vi "Read Address.vi"(8 "error in":errorcluster, 11 "Node in":refnum<class "Node.lvclass">) -> (0 "error out":errorcluster, 2 "Address":i32[](array[numeric]), 3 "Node out":refnum<class "Node.lvclass">)   [LabVIEW 2014, in "Node.lvclass"]
uses:
  Node.lvclass
  Node.lvclass/Node.ctl
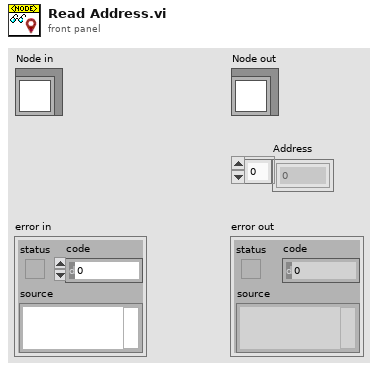
[diagram p1: front panel]
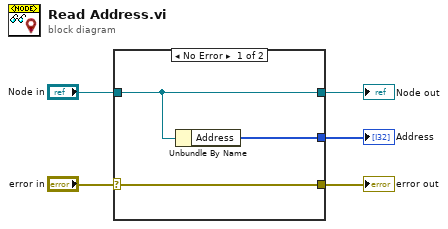
[diagram p0: block diagram]
diagram:
  n1 = case shown="No Error" "error in" {
    selector: "error in" -> [w8 w9]
    tunnel: [w8 w9] -> w4
    tunnel: [w7 w10] -> w2
    tunnel: "Node in" -> [w7 w10]
    tunnel: [w6 _] -> w1
    frame No Error {
      n2 = Unbundle By Name(w7) -> ("Address"=w6:i32[])
    }
    frame Error {
    }
  }
  "error out" <- w4
  "Node out" <- w2
  "Address" <- w1
